vi "sub1.vi"(10 "Numeric 3":i32, 11 "Numeric in":i32) -> (3 "Numeric out":i32)   [LabVIEW 2020]
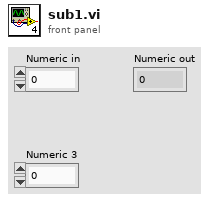
[diagram p1: front panel]
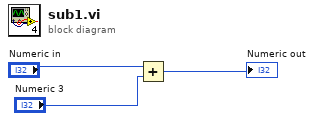
[diagram p0: block diagram]
diagram:
  n1 = Add(x="Numeric in", y="Numeric 3") -> (x+y=→"Numeric out":i32)
